vi "ROI entry-Init UI elements.vi"(8 "error in (no error)":errorcluster) -> (0 "error out":errorcluster)   [LabVIEW 2020]
uses:
  Typedefs/ROI ID Enum.ctl
  ROI Entry screen/Globals/gl_ROI Entry UI globals.vi
  Global Variables/General Globals.vi
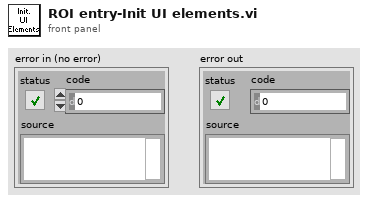
[diagram p1: front panel]
types:
  T1 = enum8{"Enabled", "Disabled", "Disabled and Grayed Out"}
  T2 = typedef "ROI ID Enum.ctl" = enum16{"Point", "MiniScan", "Comp. MiniScan", "Rectangle", "Comp. volume", "Arb. plane point", "None"}
  T3 = typedef "ROI entry screen ctrl refs cluster.ctl" = cluster{"Done button":refnum<vi>, "Imaging button":refnum<vi>, "Acquisition button":refnum<vi>, "Scan dwell time per pixel (us)":refnum<vi>, "# of planes":refnum<vi>, "Zoom Ctrl":refnum<vi>, "Equal size":refnum<vi>, "Channel":refnum<vi>, "Image Display":refnum<vi>, "Z-Plane Selector":refnum<vi>, "Number of lines left":refnum<vi>, "Z-stack folder path":refnum<vi>, "POI Density":refnum<vi>, "Arb Plane Entry":refnum<vi>, "Whole Plane":refnum<vi>, "Line Mode":refnum<vi>, "Clear Last":refnum<vi>, "Clear All":refnum<vi>, "Delete Lines":refnum<vi>, "Trial Length (sec)":refnum<vi>, "Palette Type":refnum<vi>, "Intensity slider":refnum<vi>, "# POI":refnum<vi>, "Max Z Proj":refnum<vi>, "Zplane ind":refnum<vi>, "Wavelength (nm)":refnum<vi>, "Number of Trials":refnum<vi>, "Funct stim.trig.enable":refnum<vi>, "Funct stim.trig.delay (s)":refnum<vi>, "Line Mode":refnum<vi>, "Step size (µm)":refnum<vi>, "ROI move mode":refnum<vi>, "Cool-down time (s)":refnum<vi>, "Enable cool-down time":refnum<vi>, "Motor Z ind. (um)":refnum<vi>, "AOL Z ind. (um)":refnum<vi>, "Load Reference Image":refnum<vi>, "Rel.  Res.":refnum<vi>, "ROI LIST":refnum<vi>, "Show All":refnum<vi>, "ROI Type":refnum<vi>, "Start Plane":refnum<vi>, "Stop Plane":refnum<vi>, "Offset ROI":refnum<vi>, "Tab Control":refnum<vi>, "Laser Power(%)":refnum<vi>, "Cycle rate":refnum<vi>, "FOV (Ind.)":refnum<vi>, "Frame Size (Ind.)":refnum<vi>, "Resolution (Ind.)":refnum<vi>, "Pixel Density (Ind)":refnum<vi>, "Laser Power (Ind.)":refnum<vi>, "Dwell Time (Ind.)":refnum<vi>, "Adj MC":refnum<vi>}
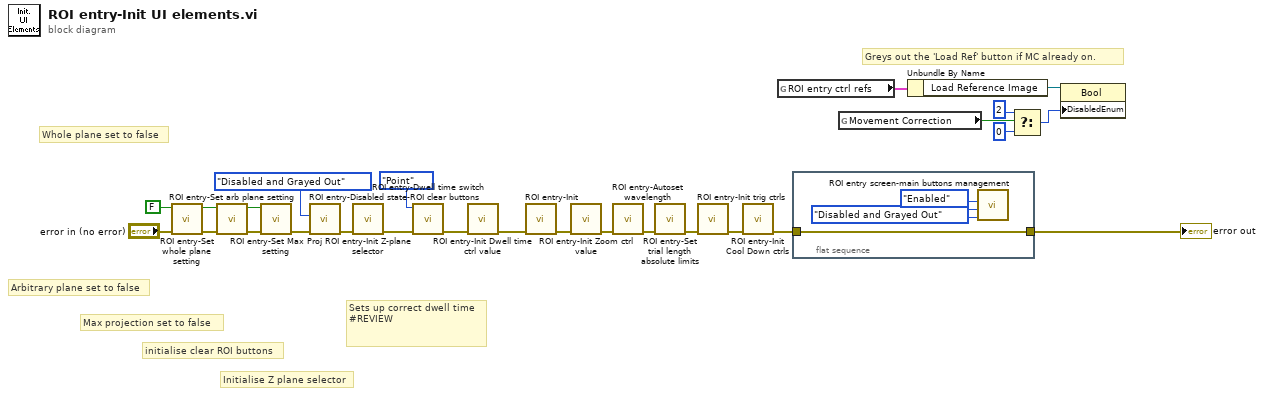
[diagram p0: block diagram]
diagram:
  w19 = FALSE ("Whole plane")
  # "Sets up correct dwell time\n#REVIEW"
  # "Initialise Z plane selector"
  # "initialise clear ROI buttons"
  # "Max projection set to false"
  # "Arbitrary plane set to false"
  # "Whole plane set to false"
  # "Greys out the 'Load Ref' button if MC already on."
  n1 = call "ROI entry-Set whole plane setting.vi"("error in (no error)"="error in (no error)", "\"Whole plane\" button's value"=w19) -> ("error out"=w20:errorcluster)  [unwired: 9 in]
  n2 = call "ROI entry-Set arb plane setting.vi"("error in (no error)"=w20, "\"Arb plane entry\" button's value"=w19) -> ("error out"=w18:errorcluster)  [unwired: 9 in]
  n3 = call "ROI entry-Set Max Proj setting.vi"("error in (no error)"=w18, "Max Z-projection button value"=w19) -> ("error out"=w21:errorcluster)  [unwired: 9 in]
  n4 = call "ROI entry-Disabled state-ROI clear buttons.vi"("error in (no error)"=w21, "State"=T1."Disabled and Grayed Out" ("Disabled")) -> ("error out"=w17:errorcluster)  [unwired: 9 in]
  n5 = call "ROI entry-Init Z-plane selector.vi"("error in (no error)"=w17) -> ("error out"=w13:errorcluster)  [unwired: 10 in]
  n6 = call "ROI entry-Dwell time switch.vi"("error in (no error)"=w13, "ROI Enum"=ROI_ID_Enum."Point") -> ("error out"=w2:errorcluster)  [unwired: 9 in]
  n7 = call "ROI entry-Init Dwell time ctrl value.vi"("error in (no error)"=w2) -> ("error out"=w1:errorcluster)  [unwired: 9 in, 1 out]
  n8 = call "ROI entry-Init.vi"("error in (no error)"=w1) -> ("error out"=w3:errorcluster)  [unwired: 10 in]
  n9 = call "ROI entry-Init Zoom ctrl value.vi"("error in (no error)"=w3) -> ("error out"=w22:errorcluster)  [unwired: 9 in, 1 out]
  n10 = call "ROI entry-Autoset wavelength.vi"("error in (no error)"=w22) -> ("error out"=w14:errorcluster)  [unwired: 10 in]
  n11 = call "ROI entry-Set trial length absolute limits.vi"("error in (no error)"=w14) -> ("error out"=w12:errorcluster)  [unwired: 10 in]
  n12 = call "ROI entry-Init trig ctrls.vi"("error in (no error)"=w12) -> ("error out"=w11:errorcluster)  [unwired: 10 in]
  n13 = call "ROI entry-Init Cool Down ctrls.vi"("error in (no error)"=w11) -> ("error out"=w10:errorcluster)  [unwired: 10 in]
  n14 = global read "gl_ROI Entry UI globals.vi" "ROI entry ctrl refs"() -> (w9:T3)
  n15 = flat-sequence {
    tunnel: w10 -> [w25]
    tunnel: [w25] -> w24
    frame #0 {
      w27 = T1."Disabled and Grayed Out" ("Disabled")
      n16 = call "ROI entry screen-main buttons management.vi"("Imaging button disabled?"=w27, "Acquisition button disabled?"=w27, "Done button disabled?"=T1."Enabled" ("Disabled")) -> ()  [unwired: 9 in]
    }
  }
  n17 = global read "General Globals.vi" "Movement Correction"() -> (w7:bool)
  n18 = Unbundle By Name(w9) -> ("Load Reference Image"=w8:refnum<vi>)
  n19 = Select(t=2, s=w7, f=0) -> (s? t:f=w6:i32)
  n20 = property class="Bool"(reference=w8, "DisabledEnum"=w6) -> ()  [unwired: 1 in, 2 out]
  "error out" <- w24
